vi "Close.vi"(8 "error in (no error)":errorcluster, 11 "CONTROLLER in":refnum<class "CONTROLLER.lvclass">) -> (0 "error out":errorcluster, 3 "CONTROLLER out":refnum<class "CONTROLLER.lvclass">)   [LabVIEW 2013, in "CONTROLLER.lvclass"]
uses:
  CONTROLLER.lvclass
  CONTROLLER.lvclass/CONTROLLER.ctl
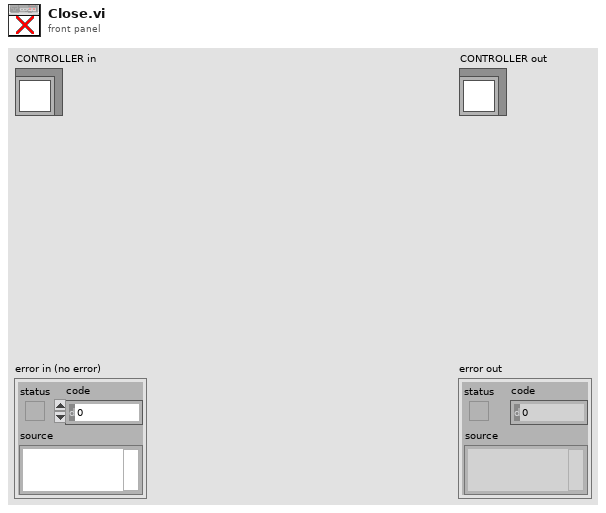
[diagram p1: front panel]
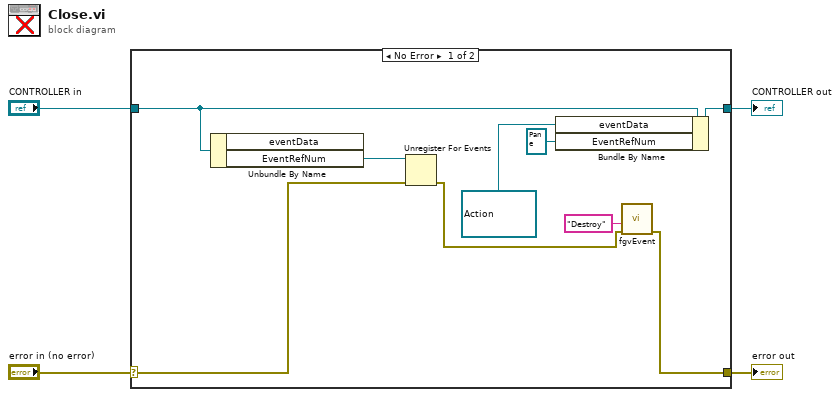
[diagram p0: block diagram]
diagram:
  n1 = case shown="No Error" "error in (no error)" {
    selector: "error in (no error)" -> [w11 w15]
    tunnel: [w5 w15] -> w3
    tunnel: [w10 w14] -> w1
    tunnel: "CONTROLLER in" -> [w13 w14]
    frame No Error {
      n2 = Unbundle By Name(w13) -> ("EventRefNum"=w12:refnum<event-registration>)  [unwired: 1 out]
      n3 = Unregister For Events(event registration refnum=w12, error in=w11) -> (error out=w6:errorcluster)
      n4 = Bundle By Name(cluster=w13, "eventData"=refnum<user-event> refnum ("ViewEvent.eventData"), "EventRefNum"=refnum<event-registration> refnum ("ViewEvent.EventRefNum")) -> (w10:refnum<class "CONTROLLER.lvclass">)
      n5 = call "fgvEvent.vi"("error in (no error)"=w6, "Cmd"="Destroy") -> ("error out"=w5:errorcluster)  [unwired: 7 in, 2 out]
    }
    frame Error {
    }
  }
  "error out" <- w3
  "CONTROLLER out" <- w1
